vi "Stop Core.vi"(10 "final error code":i32, 11 "Nested in":refnum<class "Normal Log.lvclass">) -> (3 "Nested out":refnum<class "Normal Log.lvclass">)   [LabVIEW 2020, in "Normal Log.lvlib" / "Normal Log.lvclass"]
doc: "(<B>Filename</B>: Actor Framework.lvlib:Actor.lvclass:Stop Core.vi)\n\nDefines what the actor does before it stops. Use the <B>final error code</B> input to determine whether the actor shut down in response to an error.\n\nBy default, this method does nothing. A descendant class may override it to define behavior, such as shutting down any processes the actor initiated in its override of the Actor Core method."
uses:
  Normal Log.lvclass
  Log/Log/Log.lvclass
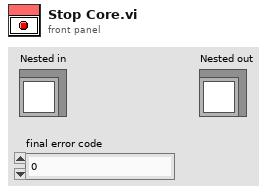
[diagram p1: front panel]
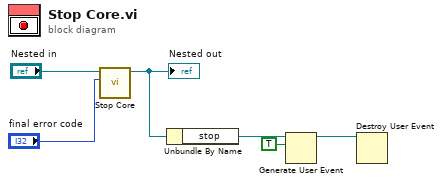
[diagram p0: block diagram]
diagram:
  n1 = call-parent "Stop Core.vi"("final error code"="final error code", "Log in"="Nested in") -> ("Log out"=w1:refnum<class "Normal Log.lvclass">)  [unwired: 9 in]
  "Nested out" <- w1
  n2 = Unbundle By Name ("Unbundle Events")(w1) -> ("stop"=w2:refnum<user-event>)
  n3 = Generate User Event(user event=w2, event data cluster=TRUE ("event data")) -> (user event out=w3:refnum<user-event>)  [unwired: 2 in, 1 out]
  n4 = Destroy User Event(user event=w3) -> ()  [unwired: 1 in, 1 out]
